vi "Aufnahme_Lichtgitter.vi"(8 "Fehler in":errorcluster, 11 "Cluster in":T1={"Initialisierung"={"Online?"=FALSE, "Grundpfad"=path "", "Kamera Oben"="", "IP-Adresse Flüssiglinse"="", "Flüssiglinse"=refnum, "Kamera Unten"="", "IP-Adresse SPS"="", "SPS-Verbindung"={"TCP Connection Ref"=refnum, "IP address"="", "timeout ms"=5000, "Connected?"=FALSE, "PLC Type"=enum."S7 1200", "Rack S7 400"=0, "Slot S7 400"=0, "PDU Size"=0, "connection semaphore"=refnum}, "IP-Adresse Lichtgitter"="", "Lichtgitter"=refnum, "Skalierungsfaktor"=0.0, "Bilder Oben"=[], "Bild Unten"=refnum, "Bild Ausschnitt Unten"=refnum}, "Einstellungen"={"Gesamtablauf gestartet"=FALSE, "i. O. Bilder speichern"=FALSE, "Bildspeicherung Offline"=FALSE, "Ausgewähltes Offline-Datum"="", "Ausgewähltes Offline-Teil"="", "Speicherpfad Bilder"=path ""}, "Artikeldaten"={"Artikelnummer"="", "Fertigungsauftrag"="", "Muster ISO"=refnum, "Belichtungszeit Referenzmarken"=0.0, "Fokus Referenzmarken"=0.0, "Belichtungszeit ISO"=0.0, "Fokus ISO"=0.0, "Belichtungszeit Unten"=0.0, "Kontaktanzahl"=0, "Aktueller Kontakt"=0, "Kontaktposition"={"x"=0.0, "y"=0.0}, "ISO-Muster nicht vorhanden"=FALSE, "Winkel ISO"=0.0, "Mittelpunkt ISO"={"x"=0.0, "y"=0.0}}, "Werte Kamera Oben"={"Koordinatensystem"={"Punkt x-Achse"={"X"=0.0, "Y"=0.0}, "Ursprung"={"X"=0.0, "Y"=0.0}, "Punkt y-Achse"={"X"=0.0, "Y"=0.0}}, "Position Kontakt"={"x"=0.0, "y"=0.0}, "Durchmesser Loch"=0.0, "Winkel Kontakt"=0.0, "Position Kontakt umgerechnet"={"x"=0.0, "y"=0.0}}, "Werte Kamera Unten"={"Prüfung Unten n. i. O."=FALSE}, "Werte Lichtgitter"={"Messwerte Referenzmarken"=[], "Mittelpunkt Referenzmarken"={"x"=0.0, "y"=0.0}, "Messwerte Kontakt"=[], "Offset"={"x"=0.0, "y"=0.0}}, "Rückmeldungen"={"Koordinaten ermittelt"=FALSE, "Vermessung Lichtgitter fertig"=FALSE, "Nachkontrolle Kamera Unten fertig"=FALSE}, "Fehler"={"Referenzen nicht gefunden"=FALSE, "Kontakt nicht gefunden"=FALSE, "Referenzen nicht in Lichtgitter"=FALSE, "Kontakt zu groß"=FALSE, "Kontakt zu klein"=FALSE}, "Statistik"={"Statistiken"=[]}, "Timer"={"Timer Start Position"=0, "Timer Start Lichtgitter"=0, "Timer Start Kamera Unten"=0}}) -> (0 "Fehler out":errorcluster, 3 "Cluster out":T1={"Initialisierung"={"Online?"=FALSE, "Grundpfad"=path "", "Kamera Oben"="", "IP-Adresse Flüssiglinse"="", "Flüssiglinse"=refnum, "Kamera Unten"="", "IP-Adresse SPS"="", "SPS-Verbindung"={"TCP Connection Ref"=refnum, "IP address"="", "timeout ms"=5000, "Connected?"=FALSE, "PLC Type"=enum."S7 1200", "Rack S7 400"=0, "Slot S7 400"=0, "PDU Size"=0, "connection semaphore"=refnum}, "IP-Adresse Lichtgitter"="", "Lichtgitter"=refnum, "Skalierungsfaktor"=0.0, "Bilder Oben"=[], "Bild Unten"=refnum, "Bild Ausschnitt Unten"=refnum}, "Einstellungen"={"Gesamtablauf gestartet"=FALSE, "i. O. Bilder speichern"=FALSE, "Bildspeicherung Offline"=FALSE, "Ausgewähltes Offline-Datum"="", "Ausgewähltes Offline-Teil"="", "Speicherpfad Bilder"=path ""}, "Artikeldaten"={"Artikelnummer"="", "Fertigungsauftrag"="", "Muster ISO"=refnum, "Belichtungszeit Referenzmarken"=0.0, "Fokus Referenzmarken"=0.0, "Belichtungszeit ISO"=0.0, "Fokus ISO"=0.0, "Belichtungszeit Unten"=0.0, "Kontaktanzahl"=0, "Aktueller Kontakt"=0, "Kontaktposition"={"x"=0.0, "y"=0.0}, "ISO-Muster nicht vorhanden"=FALSE, "Winkel ISO"=0.0, "Mittelpunkt ISO"={"x"=0.0, "y"=0.0}}, "Werte Kamera Oben"={"Koordinatensystem"={"Punkt x-Achse"={"X"=0.0, "Y"=0.0}, "Ursprung"={"X"=0.0, "Y"=0.0}, "Punkt y-Achse"={"X"=0.0, "Y"=0.0}}, "Position Kontakt"={"x"=0.0, "y"=0.0}, "Durchmesser Loch"=0.0, "Winkel Kontakt"=0.0, "Position Kontakt umgerechnet"={"x"=0.0, "y"=0.0}}, "Werte Kamera Unten"={"Prüfung Unten n. i. O."=FALSE}, "Werte Lichtgitter"={"Messwerte Referenzmarken"=[], "Mittelpunkt Referenzmarken"={"x"=0.0, "y"=0.0}, "Messwerte Kontakt"=[], "Offset"={"x"=0.0, "y"=0.0}}, "Rückmeldungen"={"Koordinaten ermittelt"=FALSE, "Vermessung Lichtgitter fertig"=FALSE, "Nachkontrolle Kamera Unten fertig"=FALSE}, "Fehler"={"Referenzen nicht gefunden"=FALSE, "Kontakt nicht gefunden"=FALSE, "Referenzen nicht in Lichtgitter"=FALSE, "Kontakt zu groß"=FALSE, "Kontakt zu klein"=FALSE}, "Statistik"={"Statistiken"=[]}, "Timer"={"Timer Start Position"=0, "Timer Start Lichtgitter"=0, "Timer Start Kamera Unten"=0}})   [LabVIEW 2024]
doc: "Überprüft ob die richtige Anzahl an Kanten in den Lichtgittern vorhanden sind und schreibt alle Messwerte in das Cluster."
uses:
  Typdefinitionen/Cluster.ctl
  <vilib>/userDefined/High Color/IMAQdx.ctl
  <vilib>/DATA AHEAD/SP7/typedefs/S7 Connection.ctl
  <vilib>/DATA AHEAD/SP7/typedefs/PLC Type.ctl
  <vilib>/vision/Image Controls.llb/IMAQ Image.ctl
  Typdefinitionen/Koordinatensystem.ctl
  Typdefinitionen/Statistik.ctl
  <vilib>/Utility/file.llb/Read Delimited Spreadsheet (DBL).vi
  <vilib>/DATA AHEAD/SP7/SP7.lvlib
panel:
  out "Lese- und Schreibestrings":string
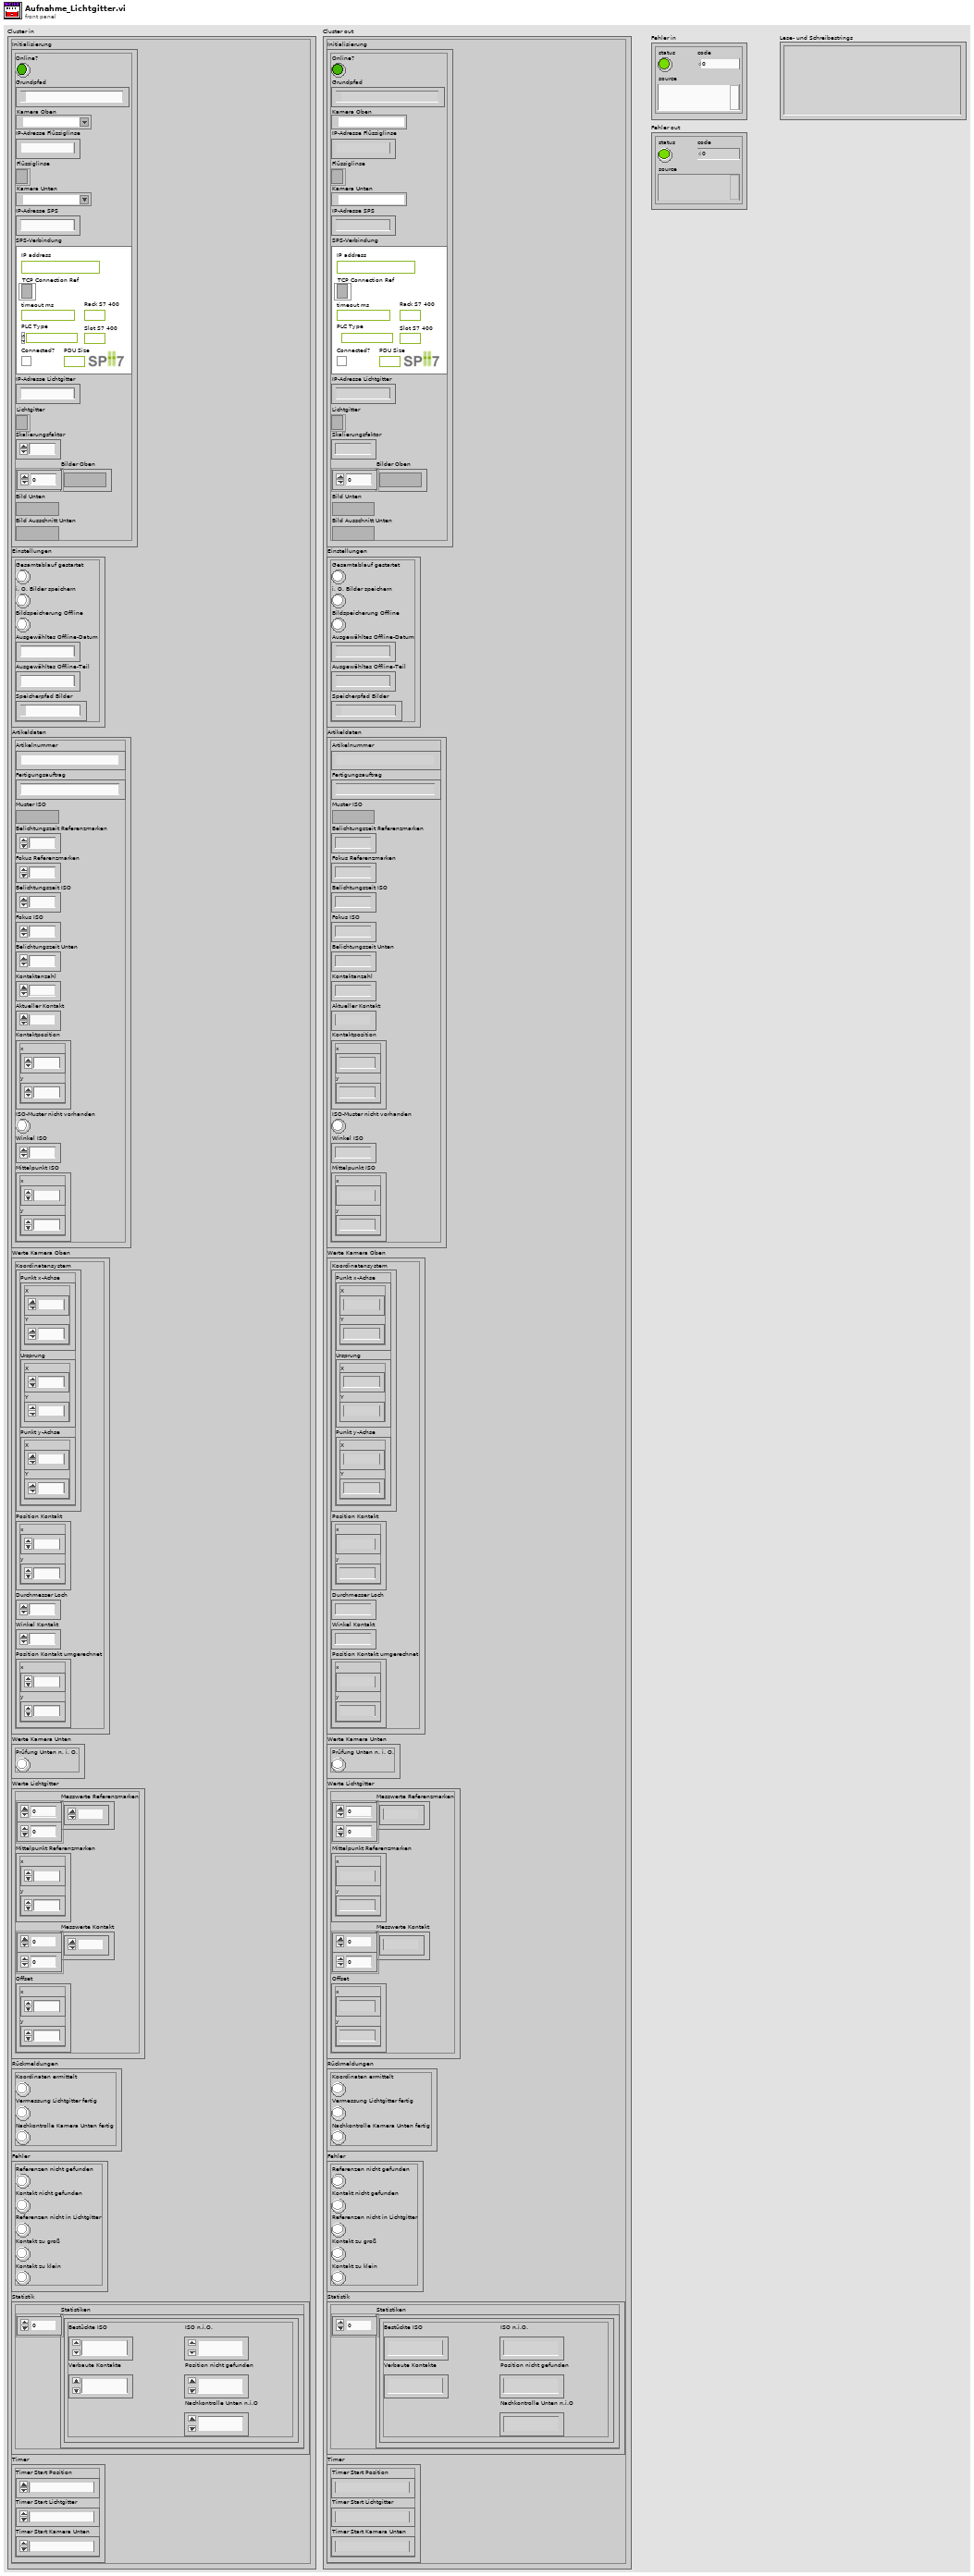
[diagram p1: front panel]
types:
  T1 = typedef "Cluster.ctl" = cluster{"Initialisierung":cluster{"Online?":bool, "Grundpfad":path, "Kamera Oben":T2, "IP-Adresse Flüssiglinse":string, "Flüssiglinse":refnum<k5>, "Kamera Unten":T2, "IP-Adresse SPS":string, "SPS-Verbindung":T3, "IP-Adresse Lichtgitter":string, "Lichtgitter":refnum<k5>, "Skalierungsfaktor":dbl, "Bilder Oben":T6[], "Bild Unten":T6, "Bild Ausschnitt Unten":T6}, "Einstellungen":cluster{"Gesamtablauf gestartet":bool, "i. O. Bilder speichern":bool, "Bildspeicherung Offline":bool, "Ausgewähltes Offline-Datum":string, "Ausgewähltes Offline-Teil":string, "Speicherpfad Bilder":path}, "Artikeldaten":cluster{"Artikelnummer":string, "Fertigungsauftrag":string, "Muster ISO":T6, "Belichtungszeit Referenzmarken":dbl, "Fokus Referenzmarken":dbl, "Belichtungszeit ISO":dbl, "Fokus ISO":dbl, "Belichtungszeit Unten":dbl, "Kontaktanzahl":u32, "Aktueller Kontakt":i16, "Kontaktposition":cluster{"x":sgl, "y":sgl}, "ISO-Muster nicht vorhanden":bool, "Winkel ISO":sgl, "Mittelpunkt ISO":cluster{"x":dbl, "y":dbl}}, "Werte Kamera Oben":cluster{"Koordinatensystem":T7, "Position Kontakt":cluster{"x":dbl, "y":dbl}, "Durchmesser Loch":dbl, "Winkel Kontakt":dbl, "Position Kontakt umgerechnet":cluster{"x":dbl, "y":dbl}}, "Werte Kamera Unten":cluster{"Prüfung Unten n. i. O.":bool}, "Werte Lichtgitter":cluster{"Messwerte Referenzmarken":dbl[][], "Mittelpunkt Referenzmarken":cluster{"x":dbl, "y":dbl}, "Messwerte Kontakt":dbl[][], "Offset":cluster{"x":dbl, "y":dbl}}, "Rückmeldungen":cluster{"Koordinaten ermittelt":bool, "Vermessung Lichtgitter fertig":bool, "Nachkontrolle Kamera Unten fertig":bool}, "Fehler":cluster{"Referenzen nicht gefunden":bool, "Kontakt nicht gefunden":bool, "Referenzen nicht in Lichtgitter":bool, "Kontakt zu groß":bool, "Kontakt zu klein":bool}, "Statistik":cluster{"Statistiken":T8[]}, "Timer":cluster{"Timer Start Position":u32, "Timer Start Lichtgitter":u32, "Timer Start Kamera Unten":u32}}
  T2 = typedef "IMAQdx.ctl" = refnum<k21>
  T3 = typedef "SP7.lvlib/S7 Connection.ctl" = cluster{"TCP Connection Ref":refnum<k5>, "IP address":string, "timeout ms":i32, "Connected?":bool, "PLC Type":T4, "Rack S7 400":u8, "Slot S7 400":u8, "PDU Size":u16, "connection semaphore":T5}
  T4 = typedef "SP7.lvlib/PLC Type.ctl" = enum16{"S7 200", "S7 300/400", "S7 1200", "S7 1500", "LOGO!8"}
  T5 = typedef "Semaphore RefNum" = refnum<k1>
  T6 = typedef "IMAQ Image.ctl" = refnum<image>
  T7 = typedef "Koordinatensystem.ctl" = cluster{"Punkt x-Achse":cluster{"X":sgl, "Y":sgl}, "Ursprung":cluster{"X":sgl, "Y":sgl}, "Punkt y-Achse":cluster{"X":sgl, "Y":sgl}}
  T8 = typedef "Statistik.ctl" = cluster{"Bestückte ISO":u32, "Verbaute Kontakte":u32, "ISO n.i.O.":u32, "Nachkontrolle Unten n.i.O":u32, "Position nicht gefunden":u32}
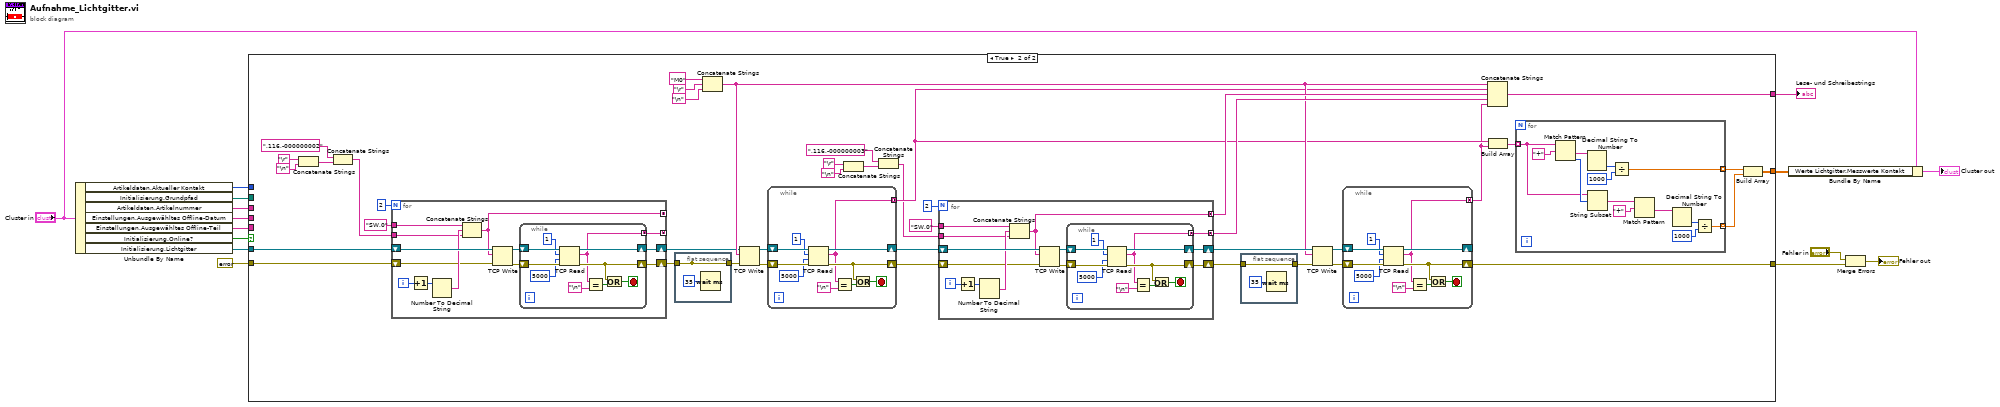
[diagram p0: block diagram]
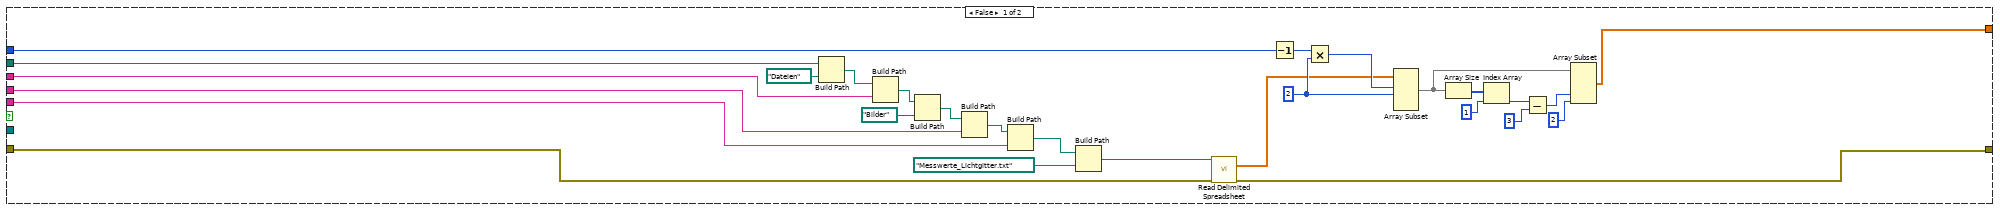
[diagram p2: hidden frame]
diagram:
  n1 = Unbundle By Name("Cluster in") -> ("Artikeldaten.Aktueller Kontakt"=w2:i16, "Initialisierung.Grundpfad"=w5:path, "Artikeldaten.Artikelnummer"=w4:string, "Einstellungen.Ausgewähltes Offline-Datum"=w6:string, "Einstellungen.Ausgewähltes Offline-Teil"=w7:string, "Initialisierung.Online?"=w8:bool, "Initialisierung.Lichtgitter"=w11:refnum<k5>)
  n2 = case shown="True" w8 {
    tunnel: [_ w84] -> w13
    tunnel: [w35 w65] -> w12
    tunnel: w11 -> [_ w59]
    tunnel: [w21 w61] -> w1
    tunnel: w7 -> [w40 _]
    tunnel: w5 -> [w29 _]
    tunnel: w6 -> [w41 _]
    tunnel: w4 -> [w26 _]
    tunnel: errorcluster {"status"=FALSE, "code"=0, "source"=""} ("Fehler in 2") -> [w36 w60]
    tunnel: w2 -> [w34 _]
    frame False {
      w32 = 2 ("length")
      n3 = Build Path(base path=w29, name or relative path=path "Dateien") -> (appended path=w28:path)
      n4 = Build Path(base path=w28, name or relative path=w26) -> (appended path=w43:path)
      n5 = Build Path(base path=w43, name or relative path=path "Bilder") -> (appended path=w30:path)
      n6 = Build Path(base path=w30, name or relative path=w41) -> (appended path=w42:path)
      n7 = Build Path(base path=w42, name or relative path=w40) -> (appended path=w39:path)
      n8 = Build Path(base path=w39, name or relative path=path "Messwerte_Lichtgitter.txt") -> (appended path=w37:path)
      n9 = call-poly <vilib>:"Read Delimited Spreadsheet.vi"("file path (dialog if empty)"=w37, "error in (no error)"=w36) -> ("all rows"=w20:dbl[][], "error out"=w35:errorcluster)  [unwired: 8 in, 4 out]
      n10 = Decrement(x=w34) -> (x-1=w33:i16)
      n11 = Multiply(x=w33, y=w32) -> (x*y=w31:i32)
      n12 = Array Subset(array=w20, index (row)=w31, length (row)=w32) -> (w22:dbl[][])  [unwired: 2 in]
      n13 = Array Size(array=w22) -> (size(s)=w24:i32[])
      n14 = Index Array(array=w24, index=1) -> (element=w19:i32)
      n15 = Subtract(x=w19, y=3) -> (x-y=w17:i32)
      n16 = Array Subset(array=w22, index (col)=w17, length (col)=2 ("length")) -> (w21:dbl[][])  [unwired: 2 in]
    }
    frame True {
      n17 = Concatenate Strings("\r", "\n") -> (w54:string)
      n18 = Concatenate Strings(",116,-000000002" ("string"), w54) -> (w49:string)
      n19 = for {
        N: 2 -> [_]
        tunnel: "SW,0" ("string") -> [w138]
        shift-right: [w141] -> w58
        shift-left: w59 -> [w139]
        shift-right: [w140] -> w57
        shift-left: w60 -> [w135]
        tunnel: w49 -> [w136]
        tunnel: [w134] -> _ mode=concatenating
        tunnel: [w133] -> _ mode=concatenating
        i -> [w143]
        n20 = Increment(x=w143) -> (x+1=w142:i32)
        n21 = Number To Decimal String(number=w142) -> (decimal integer string=w137:string)  [unwired: 1 in]
        n22 = Concatenate Strings(w138, w137, w136) -> (w133:string)
        n23 = TCP Write(connection ID=w139, data in=w133, error in (no error)=w135) -> (connection ID out=w144:refnum<k5>, error out=w145:errorcluster)  [unwired: 1 in, 1 out]
        n24 = while {
          shift-right: [w153] -> w141
          shift-left: w144 -> [w155]
          shift-right: [w149] -> w140
          shift-left: w145 -> [w154]
          tunnel: [w146] -> w134 mode=concatenating
          stop <- w148 stop-if-true
          n25 = TCP Read(connection ID=w155, bytes to read=1, error in (no error)=w154, 9:5000 ("timeout ms (25000)")) -> (connection ID out=w153:refnum<k5>, data out=w146:string, error out=w149:errorcluster)  [unwired: 1 in]
          n26 = Equal?(x=w146, y="\n") -> (x = y?=w150:bool)
          n27 = Or(x=w149, y=w150) -> (x .or. y?=w148:bool)
        }
      }
      n28 = flat-sequence {
        tunnel: w57 -> [w86]
        tunnel: [w86] -> _
        tunnel: [w86] -> w56
        frame #0 {
          n29 = Wait (ms)(milliseconds to wait=u32 35) -> ()  [unwired: 1 out]
        }
      }
      n30 = Concatenate Strings("M0" ("string"), "\r", "\n") -> (w68:string)
      n31 = TCP Write(connection ID=w58, data in=w68, error in (no error)=w56) -> (connection ID out=w79:refnum<k5>, error out=w80:errorcluster)  [unwired: 1 in, 1 out]
      n32 = while {
        shift-right: [w130] -> w76
        shift-left: w79 -> [w132]
        shift-right: [w126] -> w77
        shift-left: w80 -> [w131]
        tunnel: [w123] -> w67 mode=concatenating
        stop <- w125 stop-if-true
        n33 = TCP Read(connection ID=w132, bytes to read=1, error in (no error)=w131, 9:5000 ("timeout ms (25000)")) -> (connection ID out=w130:refnum<k5>, data out=w123:string, error out=w126:errorcluster)  [unwired: 1 in]
        n34 = Equal?(x=w123, y="\n") -> (x = y?=w127:bool)
        n35 = Or(x=w126, y=w127) -> (x .or. y?=w125:bool)
      }
      n36 = Concatenate Strings("\r", "\n") -> (w46:string)
      n37 = Concatenate Strings(",116,-000000003" ("string"), w46) -> (w44:string)
      n38 = for {
        N: 2 -> [_]
        tunnel: "SW,0" ("string") -> [w105]
        shift-right: [w108] -> w70
        shift-left: w76 -> [w106]
        shift-right: [w107] -> w71
        shift-left: w77 -> [w102]
        tunnel: w44 -> [w103]
        tunnel: [w101] -> w75 mode=concatenating
        tunnel: [w100] -> w74 mode=concatenating
        i -> [w110]
        n39 = Increment(x=w110) -> (x+1=w109:i32)
        n40 = Number To Decimal String(number=w109) -> (decimal integer string=w104:string)  [unwired: 1 in]
        n41 = Concatenate Strings(w105, w104, w103) -> (w100:string)
        n42 = TCP Write(connection ID=w106, data in=w100, error in (no error)=w102) -> (connection ID out=w111:refnum<k5>, error out=w112:errorcluster)  [unwired: 1 in, 1 out]
        n43 = while {
          shift-right: [w120] -> w108
          shift-left: w111 -> [w122]
          shift-right: [w116] -> w107
          shift-left: w112 -> [w121]
          tunnel: [w113] -> w101 mode=concatenating
          stop <- w115 stop-if-true
          n44 = TCP Read(connection ID=w122, bytes to read=1, error in (no error)=w121, 9:5000 ("timeout ms (25000)")) -> (connection ID out=w120:refnum<k5>, data out=w113:string, error out=w116:errorcluster)  [unwired: 1 in]
          n45 = Equal?(x=w113, y="\n") -> (x = y?=w117:bool)
          n46 = Or(x=w116, y=w117) -> (x .or. y?=w115:bool)
        }
      }
      n47 = flat-sequence {
        tunnel: w71 -> [w88]
        tunnel: [w88] -> w69
        frame #0 {
          n48 = Wait (ms)(milliseconds to wait=u32 35) -> ()  [unwired: 1 out]
        }
      }
      n49 = TCP Write(connection ID=w70, data in=w68, error in (no error)=w69) -> (connection ID out=w73:refnum<k5>, error out=w72:errorcluster)  [unwired: 1 in, 1 out]
      n50 = while {
        shift-right: [w97] -> _
        shift-left: w73 -> [w99]
        shift-right: [w93] -> w65
        shift-left: w72 -> [w98]
        tunnel: [w90] -> w64 mode=concatenating
        stop <- w92 stop-if-true
        n51 = TCP Read(connection ID=w99, bytes to read=1, error in (no error)=w98, 9:5000 ("timeout ms (25000)")) -> (connection ID out=w97:refnum<k5>, data out=w90:string, error out=w93:errorcluster)  [unwired: 1 in]
        n52 = Equal?(x=w90, y="\n") -> (x = y?=w94:bool)
        n53 = Or(x=w93, y=w94) -> (x .or. y?=w92:bool)
      }
      n54 = Concatenate Strings(w68, w67, w74, w75, w64) -> (w84:string)
      n55 = Build Array(w67, w64) -> (w66:string[])
      n56 = for {
        tunnel: w66 -> [w158] mode=indexing
        tunnel: [w157] -> w63 mode=indexing
        tunnel: [w156] -> w62 mode=indexing
        n57 = Match Pattern(string=w158, regular expression="+") -> (after substring=w167:string, offset past match=w159:i32)  [unwired: 1 in, 2 out]
        n58 = Decimal String To Number(string=w167) -> (number=w168:i32)  [unwired: 2 in, 1 out]
        n59 = String Subset(string=w158, offset (0)=w159) -> (substring=w164:string)  [unwired: 1 in]
        n60 = Divide(x=w168, y=1000) -> (x/y=w157:dbl)
        n61 = Match Pattern(string=w164, regular expression="+") -> (after substring=w160:string)  [unwired: 1 in, 3 out]
        n62 = Decimal String To Number(string=w160) -> (number=w161:i32)  [unwired: 2 in, 1 out]
        n63 = Divide(x=w161, y=1000) -> (x/y=w156:dbl)
      }
      n64 = Build Array(w63, w62) -> (w61:dbl[][])
    }
  }
  "Lese- und Schreibestrings" <- w13
  n65 = Bundle By Name(cluster="Cluster in", "Werte Lichtgitter.Messwerte Kontakt"=w1) -> (→"Cluster out":T1)
  n66 = Merge Errors("Fehler in", w12) -> (→"Fehler out":errorcluster)
